vi "RSZVB Get UI Data.vi"(8 "error in (no error)":errorcluster {"code" format="%.0x"}, 9 "Port (A)":i32(ring) items=["A", "B", "C", "D", "E", "F"], 11 "VISA session":refnum<visa-resource-name>) -> (0 "error out":errorcluster {"code" format="%.0x"}, 2 "Data":i32, 3 "dup VISA session":refnum<visa-resource-name>)   [LabVIEW 2011]
doc: "This VI reads data from ports A, B, C, D, E, F. If the port is an output port, the queries return the last value that was written to the port.\n\nRemote-control command(s):\nCONTrol:HANDler:A[:DATA]?\nCONTrol:HANDler:B[:DATA]?\nCONTrol:HANDler:C[:DATA]?\nCONTrol:HANDler:D[:DATA]?\nCONTrol:HANDler:E[:DATA]?\nCONTrol:HANDler:F[:DATA]?"
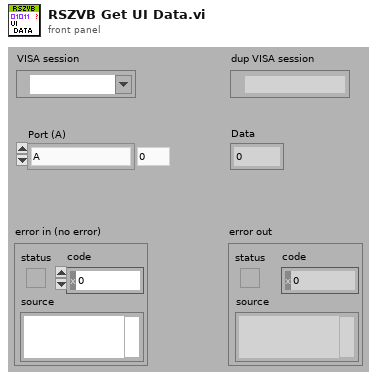
[diagram p1: front panel]
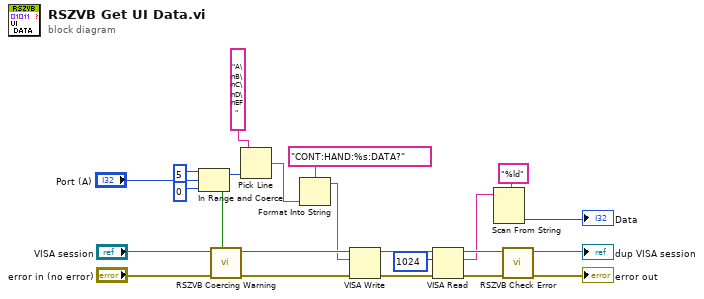
[diagram p0: block diagram]
diagram:
  n1 = In Range and Coerce(upper limit=5, x="Port (A)", lower limit=0) -> (coerced(x)=w11:i32, In Range?=w12:bool)
  n2 = call "RSZVB Coercing Warning.vi"("In Range?"=w12, "error in (no error)"="error in (no error)", "VISA session"="VISA session") -> ("error out"=w15:errorcluster, "dup VISA session"=w14:refnum<visa-resource-name>)  [unwired: 7 in]
  n3 = Pick Line(multi-line string="A\nB\nC\nD\nEF", line index=w11) -> (output string=w10:string)  [unwired: 1 in]
  n4 = Format Into String(format string="CONT:HAND:%s:DATA?", w10) -> (resulting string=w13:string)  [unwired: 2 in, 1 out]
  n5 = VISA Write(VISA resource name=w14, write buffer=w13, error in (no error)=w15) -> (VISA resource name out=w21:refnum<visa-resource-name>, error out=w23:errorcluster)  [unwired: 1 out]
  n6 = VISA Read(VISA resource name=w21, byte count=u32 1024 ("byte count (0)"), error in (no error)=w23) -> (VISA resource name out=w20:refnum<visa-resource-name>, read buffer=w7:string, error out=w19:errorcluster)  [unwired: 1 out]
  n7 = Scan From String(format string="%ld", input string=w7) -> (output 1=→"Data":i32)  [unwired: 3 in, 3 out]
  n8 = call "RSZVB Check Error.vi"("error in (no error)"=w19, "VISA session"=w20) -> ("error out"=→"error out":errorcluster, "dup VISA session"=→"dup VISA session":refnum<visa-resource-name>)  [unwired: 8 in]
